vi "PH_VacuumControl.set Running.vi"(0 "VI in":refnum<vi>, 2 "Running":bool, 5 "error in (no error)":errorcluster) -> (14 "VI out":refnum<vi>, 19 "error out":errorcluster)   [LabVIEW 2014, in "PH_VacuumControl.lvlib"]
uses:
  PH_VacuumControl.lvlib
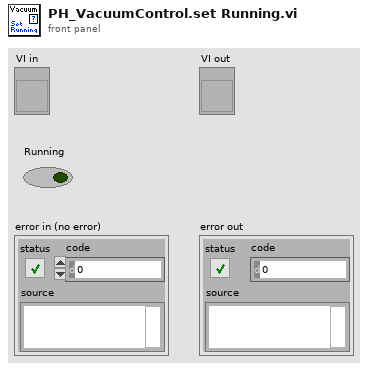
[diagram p1: front panel]
types:
  T1 = typedef "PH_VacuumControl.lvlib/PH_VacuumControl.i attribute.ctl" = cluster{"GUI Refs":cluster{"Exit":refnum<vi>, "Set Unit":refnum<vi>, "Device found":refnum<vi>, "Busy":refnum<vi>, "State":refnum<vi>, "Delete":refnum<vi>, "Channels":refnum<vi>, "Channel Name":refnum<vi>, "Trend":refnum<vi>, "Logarithmic":refnum<vi>, "Limit reached":refnum<vi>, "Channel Name 1 MT":refnum<vi>, "Channel Name 2 MT":refnum<vi>, "Trend MT":refnum<vi>, "Logarithmic MT":refnum<vi>, "Limit reached MT":refnum<vi>}, "Device found":bool, "Busy":bool, "Selected Unit":i32, "Channels [mbar]":T2, "Channel Names":cluster{"Channel 1":string, "Channel 2":string, "Channel 3":string, "Channel 4":string, "Channel 5":string, "Channel 6":string}, "Status":T3, "AGCxxx VISA Cluster":T4, "Instr Firmware Revision":string, "Service IDs Pressure":cluster{"Channel 1":i32, "Channel 2":i32, "Channel 3":i32, "Channel 4":i32, "Channel 5":i32, "Channel 6":i32}, "Service IDs Limits":cluster{"Channel 1":i32, "Channel 2":i32, "Channel 3":i32, "Channel 4":i32, "Channel 5":i32, "Channel 6":i32}, "Trend":cluster{"Start Point":timestamp, "Pressures [mbar] Channel 1":dbl[], "Pressures [mbar] Channel 2":dbl[], "Pressures [mbar] Channel 3":dbl[], "Pressures [mbar] Channel 4":dbl[], "Pressures [mbar] Channel 5":dbl[], "Pressures [mbar] Channel 6":dbl[], "Timebase [s]":i32[], "Trend Channel":u16, "Start Fit":dbl, "Trend Channel 1 MT":u16, "Trend Channel 2 MT":u16, "Start or continue Fit MT":dbl, "Continue or start Fit MT":dbl, "Datasets strored":i32, "Dataarray Size":i32}, "Running":bool}
  T2 = typedef "PH_VacuumControl.lvlib/PH_VacuumControl.Channels.ctl" = cluster{"Channel 1":dbl, "Channel 2":dbl, "Channel 3":dbl, "Channel 4":dbl, "Channel 5":dbl, "Channel 6":dbl, "Name Channel 1":string, "Name Channel 2":string, "Name Channel 3":string, "Name Channel 4":string, "Name Channel 5":string, "Name Channel 6":string, "Upper Limit":dbl, "Upper Limit 2":dbl, "Upper Limit 3":dbl, "Upper Limit 4":dbl, "Upper Limit 5":dbl, "Upper Limit 6":dbl}
  T3 = typedef "PH_StatusHandler.lvlib/PH_StatusHandler.Status.ctl" = i16
  T4 = typedef "AGCxxx - Driver.lvlib/AGCxxx VISA Control.ctl" = cluster{"VISA resource name":refnum<visa-resource-name>, "VISA Timeout Value (1000 ms)":u32, "Lock Timeout (1000 ms)":u32, "MAX Channel (6)":i32}
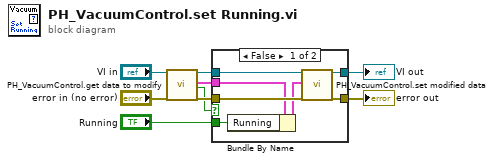
[diagram p0: block diagram]
diagram:
  n1 = call "PH_VacuumControl.get data to modify.vi"("i ref in"="VI in", "error in (no error)"="error in (no error)") -> ("i ref out"=w5:refnum<vi>, "i attribute"=w3:T1, "timed out"=w2:bool, "error out"=w8:errorcluster)  [unwired: 14 in]
  n2 = case shown="False" w2 {
    tunnel: w8 -> [w16 w17]
    tunnel: [w15 w17] -> w6
    tunnel: w5 -> [w14 w18]
    tunnel: [w13 w18] -> w4
    tunnel: w3 -> [w12 _]
    tunnel: "Running" -> [w10 _]
    frame False {
      n3 = Bundle By Name(cluster=w12, "Running"=w10) -> (w11:T1)
      n4 = call "PH_VacuumControl.set modified data.vi"("i ref in"=w14, "i attribute"=w11, "error in (no error)"=w16) -> ("i ref out"=w13:refnum<vi>, "error out"=w15:errorcluster)  [unwired: 15 in]
    }
    frame True {
    }
  }
  "VI out" <- w4
  "error out" <- w6
